vi "Right Rocket Double Level 1.vi"(11 "Level 1? (F)":bool) -> ()   [LabVIEW 2018]
uses:
  Auton Kill Switch.vi
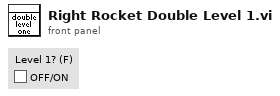
[diagram p1: front panel]
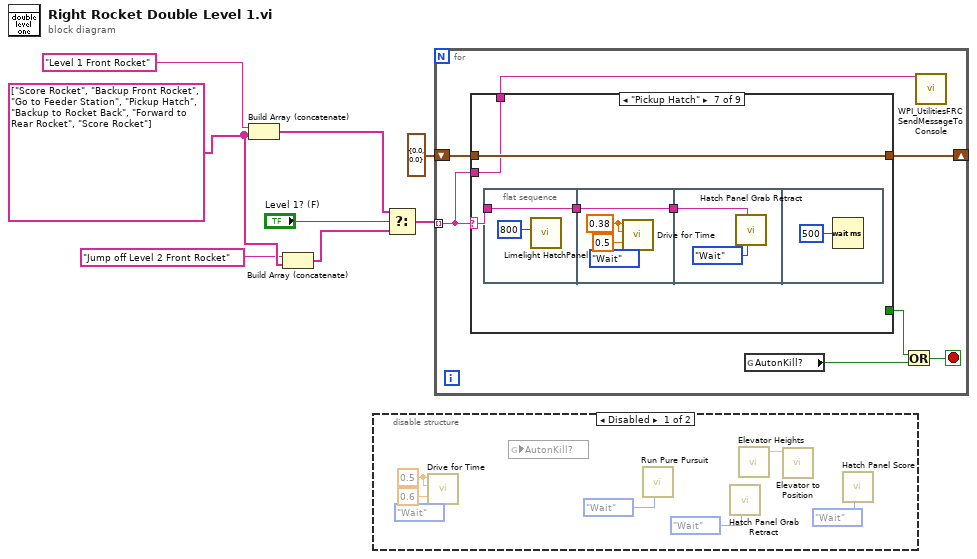
[diagram p0: block diagram]
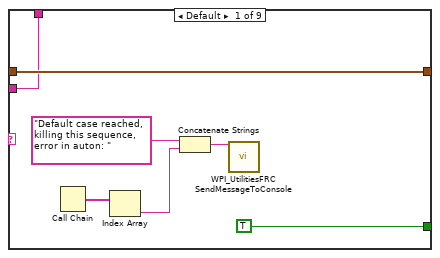
[diagram p3: hidden frame]
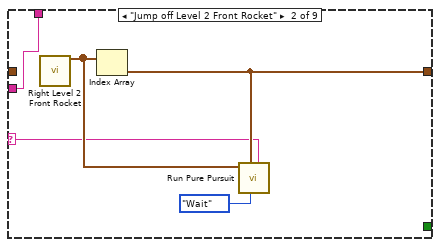
[diagram p4: hidden frame]
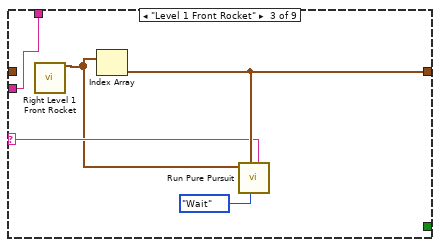
[diagram p5: hidden frame]
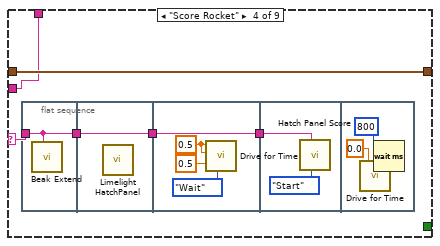
[diagram p6: hidden frame]
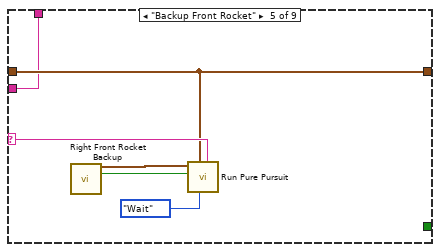
[diagram p7: hidden frame]
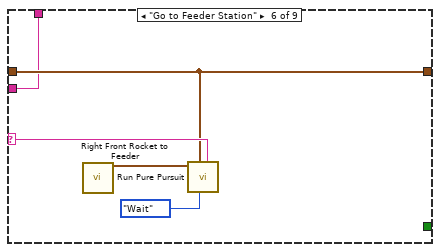
[diagram p8: hidden frame]
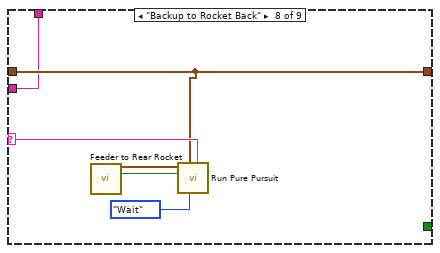
[diagram p9: hidden frame]
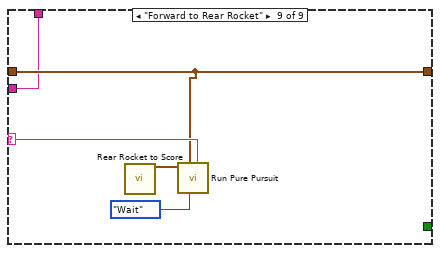
[diagram p10: hidden frame]
diagram:
  w6 = string[] ["Score Rocket", "Backup Front Rocket", "Go to Feeder Station", "Pickup Hatch", "Backup to Rocket Back", "Forward to Rear Rocket", "Score Rocket"]
  n1 = Build Array (concatenate)("Level 1 Front Rocket", w6) -> (w2:string[])
  n2 = Build Array (concatenate)("Jump off Level 2 Front Rocket", w6) -> (w3:string[])
  n3 = disable-structure shown="Disabled" {
    frame Disabled {
      w9 = 0.5 ("Left Speed")
      n4 = call "Drive for Time.vi"("Synchronization"=enum16{"Start", "Wait"}."Wait", "Seconds"=0.6, "Right Speed"=w9, "Left Speed"=w9) -> ()  [unwired: 6 in, 2 out]
      n5 = global read "Auton Kill Switch.vi" "AutonKill?"() -> ()  [unwired: 1 in]
      n6 = call "Run Pure Pursuit.vi"("Synchronication"=enum16{"Start", "Wait"}."Wait") -> ()  [unwired: 10 in, 1 out]
      n7 = call "Hatch Panel Grab Retract.vi"("Synchronization"=enum16{"Start", "Wait"}."Wait") -> ()  [unwired: 10 in, 1 out]
      n8 = call "Elevator Heights.vi"() -> ("Height"=w14:dbl)  [unwired: 9 in, 2 out]
      n9 = call "Elevator to Position.vi"("Elevator Height"=w14) -> ()  [unwired: 10 in, 1 out]
      n10 = call "Hatch Panel Score.vi"("Synchronization"=enum16{"Start", "Wait"}."Wait") -> ()  [unwired: 10 in, 1 out]
    }
    frame Enabled {
    }
  }
  n11 = Select(t=w2, s="Level 1? (F)", f=w3) -> (s? t:f=w1:string[])
  n12 = for {
    tunnel: w1 -> [w16] mode=indexing
    shift-right: [w21] -> _
    shift-left: cluster{"X":dbl, "Y":dbl} {"X"=0.0, "Y"=0.0} -> [w20]
    stop <- w19 stop-if-true
    n13 = case shown="\"Pickup Hatch\"" w16 {
      selector: w16 -> [_ w31 w37 w41 w58 w65 w70 w85 w90]
      tunnel: [w28 w32 w38 w45 w57 w64 w71 w84 w89] -> w21
      tunnel: w20 -> [w28 _ _ w45 w57 w64 w71 w84 w89]
      tunnel: [TRUE _ _ _ _ _ _ _ _] -> w18
      tunnel: [w23 w30 w36 w40 w56 w62 w69 w81 w87] -> w17
      tunnel: w16 -> [w23 w30 w36 w40 w56 w62 w69 w81 w87]
      frame Default {
        n14 = Call Chain() -> (call chain=w27:string[])
        n15 = Index Array(array=w27) -> (element=w25:string)  [unwired: 1 in]
        n16 = Concatenate Strings("Default case reached, killing this sequence, error in auton: " ("Message"), w25) -> (w24:string)
        n17 = call <vilib>:"WPI_UtilitiesFRC SendMessageToConsole.vi"("Message"=w24) -> ()  [unwired: 14 in, 1 out]
      }
      frame "Jump off Level 2 Front Rocket" {
        n18 = call "Right Level 2 Front Rocket.vi"() -> ("path"=w33:cluster{"X":dbl, "Y":dbl}[])  [unwired: 14 in, 1 out]
        n19 = Index Array(array=w33) -> (element=w32:cluster{"X":dbl, "Y":dbl})  [unwired: 1 in]
        n20 = call "Run Pure Pursuit.vi"("Description"=w31, "Synchronication"=enum16{"Start", "Wait"}."Wait", "Auton Start Point"=w32, "Path"=w33) -> ()  [unwired: 7 in, 1 out]
      }
      frame "Level 1 Front Rocket" {
        n21 = call "Right Level 1 Front Rocket.vi"() -> ("path"=w35:cluster{"X":dbl, "Y":dbl}[])  [unwired: 14 in, 1 out]
        n22 = Index Array(array=w35) -> (element=w38:cluster{"X":dbl, "Y":dbl})  [unwired: 1 in]
        n23 = call "Run Pure Pursuit.vi"("Description"=w37, "Synchronication"=enum16{"Start", "Wait"}."Wait", "Auton Start Point"=w38, "Path"=w35) -> ()  [unwired: 7 in, 1 out]
      }
      frame "Score Rocket" {
        n24 = flat-sequence {
          tunnel: w41 -> [w46]
          tunnel: [w46] -> w44
          tunnel: [w47] -> w43
          tunnel: w44 -> [w47]
          tunnel: w43 -> [w51]
          tunnel: [w51] -> w42
          tunnel: w42 -> [w52]
          frame #0 {
            n25 = call "Beak Extend.vi"("Description"=w46) -> ()  [unwired: 10 in, 1 out]
          }
          frame #1 {
            n26 = call "Limelight HatchPanel.vi"() -> ()  [unwired: 10 in, 2 out]
          }
          frame #2 {
            w50 = 0.5 ("Left Speed")
            n27 = call "Drive for Time.vi"("Synchronization"=enum16{"Start", "Wait"}."Wait", "Seconds"=0.5, "Right Speed"=w50, "Left Speed"=w50) -> ()  [unwired: 6 in, 2 out]
          }
          frame #3 {
            n28 = call "Hatch Panel Score.vi"("Synchronization"=enum16{"Start", "Wait"}."Start", "Description"=w52) -> ()  [unwired: 9 in, 1 out]
          }
          frame #4 {
            w54 = 0.0 ("Left Speed")
            n29 = call "Drive for Time.vi"("Seconds"=w54, "Right Speed"=w54, "Left Speed"=w54) -> ()  [unwired: 7 in, 2 out]
            n30 = Wait (ms)(milliseconds to wait=u32 800) -> ()  [unwired: 1 out]
          }
        }
      }
      frame "Backup Front Rocket" {
        n31 = call "Right Front Rocket Backup.vi"() -> ("path"=w60:cluster{"X":dbl, "Y":dbl}[], "Reverse Path?"=w59:bool)  [unwired: 14 in]
        n32 = call "Run Pure Pursuit.vi"("Description"=w58, "Synchronication"=enum16{"Start", "Wait"}."Wait", "Auton Start Point"=w57, "Reverse? (F)"=w59, "Path"=w60) -> ()  [unwired: 6 in, 1 out]
      }
      frame "Go to Feeder Station" {
        n33 = call "Right Front Rocket to Feeder.vi"() -> ("path"=w63:cluster{"X":dbl, "Y":dbl}[])  [unwired: 14 in, 1 out]
        n34 = call "Run Pure Pursuit.vi"("Description"=w65, "Synchronication"=enum16{"Start", "Wait"}."Wait", "Auton Start Point"=w64, "Path"=w63) -> ()  [unwired: 7 in, 1 out]
      }
      frame "Pickup Hatch" {
        n35 = flat-sequence {
          tunnel: w70 -> [w73]
          tunnel: [w73] -> w67
          tunnel: [w77] -> w68
          tunnel: w67 -> [w77]
          tunnel: w68 -> [w78]
          frame #0 {
            n36 = call "Limelight HatchPanel.vi"("Max Time ms (2000)"=u32 800) -> ()  [unwired: 9 in, 2 out]
          }
          frame #1 {
            w76 = 0.38 ("Left Speed")
            n37 = call "Drive for Time.vi"("Synchronization"=enum16{"Start", "Wait"}."Wait", "Seconds"=0.5, "Right Speed"=w76, "Left Speed"=w76) -> ()  [unwired: 6 in, 2 out]
          }
          frame #2 {
            n38 = call "Hatch Panel Grab Retract.vi"("Synchronization"=enum16{"Start", "Wait"}."Wait", "Description"=w78) -> ()  [unwired: 9 in, 1 out]
          }
          frame #3 {
            n39 = Wait (ms)(milliseconds to wait=u32 500) -> ()  [unwired: 1 out]
          }
        }
      }
      frame "Backup to Rocket Back" {
        n40 = call "Feeder to Rear Rocket.vi"() -> ("path"=w83:cluster{"X":dbl, "Y":dbl}[], "Reverse Path?"=w82:bool)  [unwired: 14 in]
        n41 = call "Run Pure Pursuit.vi"("Description"=w85, "Synchronication"=enum16{"Start", "Wait"}."Wait", "Auton Start Point"=w84, "Reverse? (F)"=w82, "Path"=w83) -> ()  [unwired: 6 in, 1 out]
      }
      frame "Forward to Rear Rocket" {
        n42 = call "Rear Rocket to Score.vi"() -> ("path"=w88:cluster{"X":dbl, "Y":dbl}[])  [unwired: 14 in, 1 out]
        n43 = call "Run Pure Pursuit.vi"("Description"=w90, "Synchronication"=enum16{"Start", "Wait"}."Wait", "Auton Start Point"=w89, "Path"=w88) -> ()  [unwired: 7 in, 1 out]
      }
    }
    n44 = global read "Auton Kill Switch.vi" "AutonKill?"() -> (w22:bool)
    n45 = Or(x=w18, y=w22) -> (x .or. y?=w19:bool)
    n46 = call <vilib>:"WPI_UtilitiesFRC SendMessageToConsole.vi"("Message"=w17) -> ()  [unwired: 14 in, 1 out]
  }
